vi "Auto Drive X.vi"(0 "PID Gains":T1={"proportional gain (Kc)"=0.07, "integral time (Ti, min)"=0.0, "derivative time (Td, min)"=0.0}, 4 "Settling Time (ms)":u32=50, 6 "Max Time (ms)":u32=15000, 8 "Min Time (ms)":u32=250, 9 "Angle to Turn (Deg)":dbl=90.0 format="%#_13g", 10 "Motor Output Range":cluster{"output high":dbl, "output low":dbl}={"output high"=0.7, "output low"=-0.7}, 11 "RobotDriveDevRef In":T2={"DevStatus"={"status"=FALSE, "code"=0, "source"=""}, "Motors[]"=[], "Square Inputs"=FALSE, "Max Output"=1.0}) -> (3 "RobotDriveDevRef Out":T2={"DevStatus"={"status"=FALSE, "code"=0, "source"=""}, "Motors[]"=[], "Square Inputs"=FALSE, "Max Output"=1.0})   [LabVIEW 2017]
uses:
  <vilib>/Rock Robotics/WPI/RobotDrive/WPI_RobotDriveDevRef.ctl
  <vilib>/Rock Robotics/WPI/MotorControl/WPI_MotorControlDeviceRef.ctl
  <vilib>/Rock Robotics/WPI/MotorControl/WPI_MotorControlType.ctl
  <vilib>/Rock Robotics/SystemInterfaces/DIO/FPGA_DIOPWMChannel.ctl
  <vilib>/Rock Robotics/WPI/PWM/WPI_PWMDeadband.ctl
  <vilib>/Rock Robotics/SystemInterfaces/DIO/FPGA_DIOChannel.ctl
  Globals/Robot Global Data.vi
  <vilib>/addons/control/pid/pid.llb/PID (DBL).vi
  <vilib>/Rock Robotics/WPI/RobotDrive/WPI_RobotDriveArcadeDrive_Standard(NoSaturation).vi
  <vilib>/addons/control/pid/NI_PID_pid.lvlib
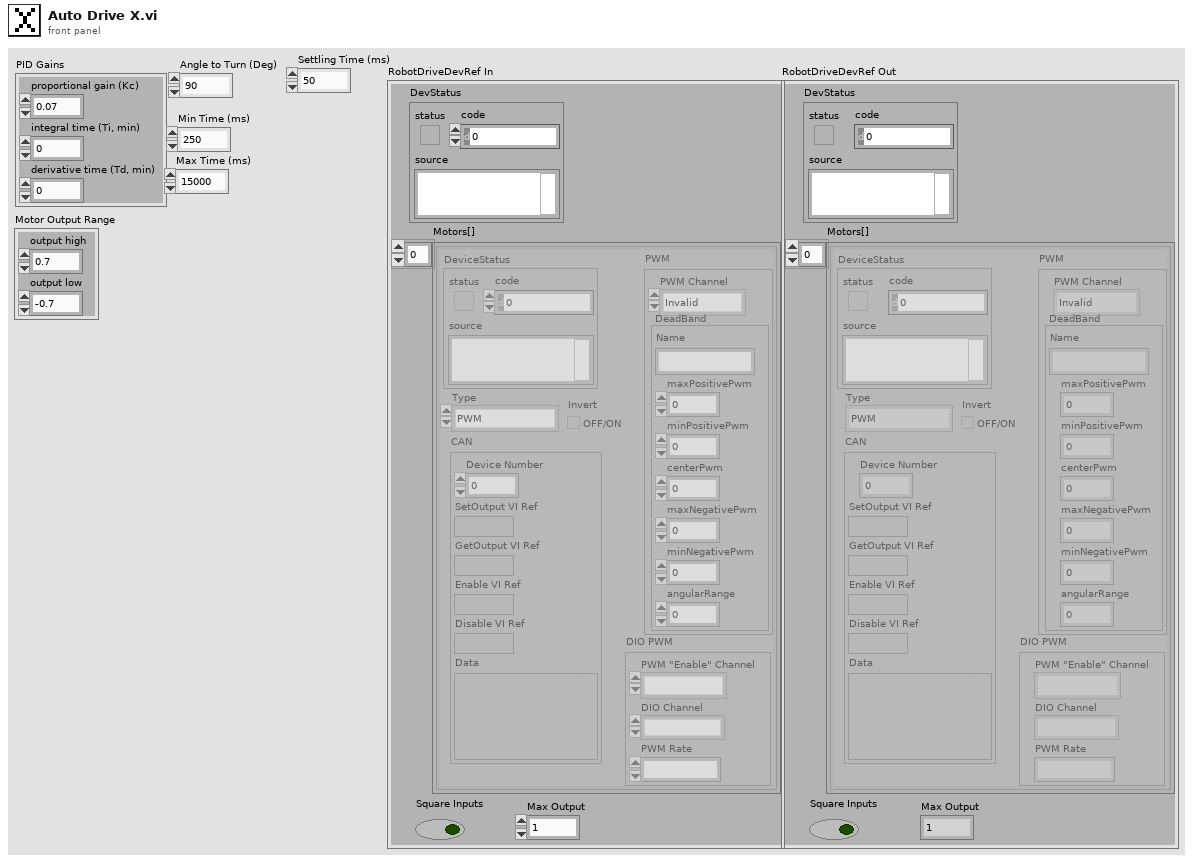
[diagram p1: front panel]
types:
  T1 = cluster{"proportional gain (Kc)":dbl, "integral time (Ti, min)":dbl, "derivative time (Td, min)":dbl}
  T2 = typedef "WPI_RobotDriveDevRef.ctl" = cluster{"DevStatus":errorcluster, "Motors[]":T3[], "Square Inputs":bool, "Max Output":dbl}
  T3 = typedef "WPI_MotorControlDeviceRef.ctl" = cluster{"DeviceStatus":errorcluster, "Type":T4, "PWM":cluster{"PWM Channel":T5, "DeadBand":T6}, "CAN":cluster{"Device Number":u8, "SetOutput VI Ref":variant, "GetOutput VI Ref":variant, "Enable VI Ref":variant, "Disable VI Ref":variant, "Data":variant}, "Invert":bool, "DIO PWM":cluster{"PWM \"Enable\" Channel":T5, "DIOChannel":T7, "PWM Rate":dbl}}
  T4 = typedef "WPI_MotorControlType.ctl" = enum16{"PWM", "CAN", "DIO PWM"}
  T5 = typedef "FPGA_DIOPWMChannel.ctl" = enum8{"PWM 0", "PWM 1", "PWM 2", "PWM 3", "PWM 4", "PWM 5", "PWM 6", "PWM 7", "PWM 8", "PWM 9", "PWM MXP 0", "PWM MXP 1", "PWM MXP 2", "PWM MXP 3", "PWM MXP 4", "PWM MXP 5", "PWM MXP 6", "PWM MXP 7", "PWM MXP 8", "PWM MXP 9", "Invalid"}
  T6 = typedef "WPI_PWMDeadband.ctl" = cluster{"Name":string, "maxPositivePwm":i32, "minPositivePwm":i32, "centerPwm":i32, "maxNegativePwm":i32, "minNegativePwm":i32, "angularRange":u16}
  T7 = typedef "FPGA_DIOChannel.ctl" = enum8{"DIO 0", "DIO 1", "DIO 2", "DIO 3", "DIO 4", "DIO 5", "DIO 6", "DIO 7", "DIO 8", "DIO 9", "DIO MXP 0", "DIO MXP 1", "DIO MXP 2", "DIO MXP 3", "DIO MXP 4", "DIO MXP 5", "DIO MXP 6", "DIO MXP 7", "DIO MXP 8", "DIO MXP 9", "DIO MXP 10", "DIO MXP 11", "DIO MXP 12", "DIO MXP 13", "DIO MXP 14", "DIO MXP 15", "SPI Port CS1", "SPI Port CS2", "SPI Port CS3", "SPI Port MISO", "SPI Port MOSI", "Invalid"}
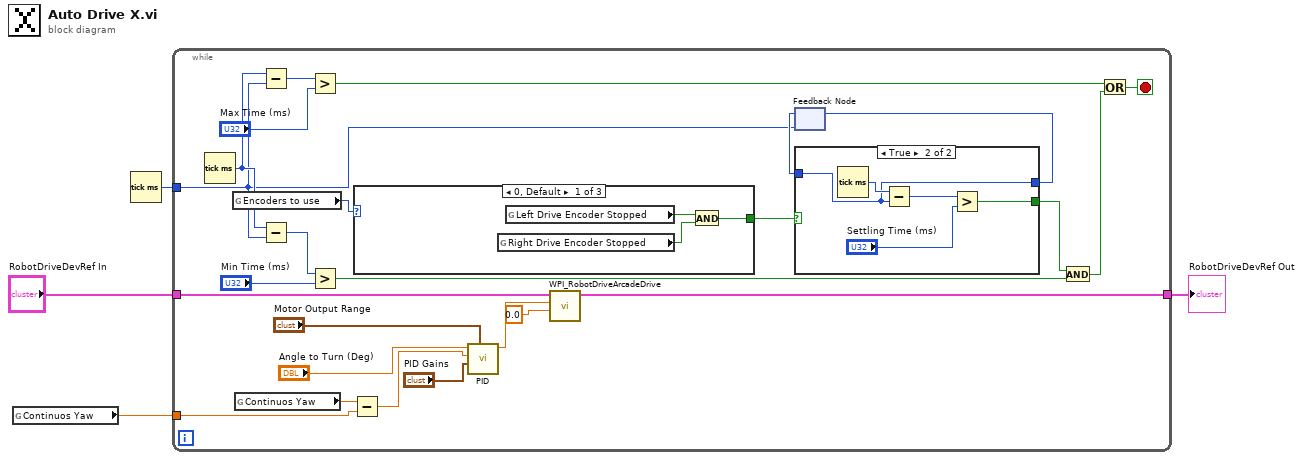
[diagram p0: block diagram]
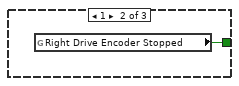
[diagram p2: hidden frame]
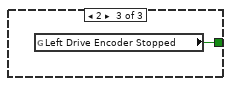
[diagram p3: hidden frame]
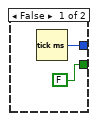
[diagram p4: hidden frame]
diagram:
  n1 = global read "Robot Global Data.vi" "Continuos Yaw"() -> (w4:dbl)
  n2 = Tick Count (ms)() -> (millisecond timer value=w3:u32)
  n3 = while {
    tunnel: "RobotDriveDevRef In" -> [w26]
    tunnel: w4 -> [w22]
    tunnel: w3 -> [w7]
    tunnel: [w18] -> w2
    stop <- w8 stop-if-true
    n4 = Tick Count (ms)() -> (millisecond timer value=w11:u32)
    n5 = global read "Robot Global Data.vi" "Encoders to use"() -> (w6:u16)
    n6 = global read "Robot Global Data.vi" "Continuos Yaw"() -> (w23:dbl)
    n7 = Subtract(x=w11, y=w7) -> (x-y=w13:u32)
    n8 = Subtract(x=w11, y=w7) -> (x-y=w17:u32)
    n9 = Greater?(x=w13, y="Max Time (ms)") -> (0:w12:bool)
    n10 = Greater?(x=w17, y="Min Time (ms)") -> (0:w15:bool)
    n11 = Subtract(x=w23, y=w22) -> (x-y=w21:dbl)
    n12 = case shown="0, Default" w6 {
      tunnel: [w32 w33 w34] -> w5
      frame 0, Default {
        n13 = global read "Robot Global Data.vi" "Right Drive Encoder Stopped"() -> (w30:bool)
        n14 = global read "Robot Global Data.vi" "Left Drive Encoder Stopped"() -> (w31:bool)
        n15 = And(x=w31, y=w30) -> (x .and. y?=w32:bool)
      }
      frame 1 {
        n16 = global read "Robot Global Data.vi" "Right Drive Encoder Stopped"() -> (w33:bool)
      }
      frame 2 {
        n17 = global read "Robot Global Data.vi" "Left Drive Encoder Stopped"() -> (w34:bool)
      }
    }
    n18 = call-poly <vilib>:"PID.vi"("output range"="Motor Output Range", "PID gains"="PID Gains", "process variable"=w21, "setpoint"="Angle to Turn (Deg)") -> ("output"=w20:dbl)  [unwired: 6 in, 1 out]
    n19 = call-poly <vilib>:"WPI_RobotDriveArcadeDrive.vi"("Y axis value"=0.0, "X axis value"=w20, "RobotDriveDevRef"=w26) -> ("RobotDriveDevRef"=w18:T2)  [unwired: 6 in, 2 out]
    n20 = feedback #1(w7) -> (w24:u32)
    n21 = case shown="True" w5 {
      tunnel: w24 -> [_ w40]
      tunnel: [w36 w40] -> w25
      tunnel: [FALSE w37] -> w10
      frame False {
        n22 = Tick Count (ms)() -> (millisecond timer value=w36:u32)
      }
      frame True {
        n23 = Tick Count (ms)() -> (millisecond timer value=w41:u32)
        n24 = Subtract(x=w41, y=w40) -> (x-y=w39:u32)
        n25 = Greater?(x=w39, y="Settling Time (ms)") -> (0:w37:bool)
      }
    }
    n26 = feedback-in #1(w25) -> ()
    n27 = And(x=w10, y=w15) -> (x .and. y?=w9:bool)
    n28 = Or(x=w12, y=w9) -> (x .or. y?=w8:bool)
  }
  "RobotDriveDevRef Out" <- w2
